vi "Title-Add.vi"(1 "Parameters":variant, 2 "String":string) -> (0 "Variant":variant)   [LabVIEW 2025]
doc: "Author: Scott Hannahs <sth@magnet.fsu.edu>\n\nThis software is licensed for use under the “MIT License\"\nCopyright (c) 2025 Scott Hannahs, sth@sth@magnet.sthnet.net\n\nPermission is hereby granted, free of charge, to any person obtaining a copy of this software and associated documentation files (the \"Software\"), to deal in the Software without restriction, including without limitation the rights to use, copy, modify, merge, publish, distribute, sublicense, and/or sell copies of the Software, and to permit persons to whom the Software is furnished to do so, subject to the following conditions: The above copyright notice and this permission notice shall be included in all copies or substantial portions of the Software.\n\nTHE SOFTWARE IS PROVIDED \"AS IS\", WITHOUT WARRANTY OF ANY KIND, EXPRESS OR IMPLIED, INCLUDING BUT NOT LIMITED TO THE WARRANTIES OF MERCHANTABILITY, FITNESS FOR A PARTICULAR PURPOSE AND NONINFRINGEMENT. IN NO EVENT SHALL THE AUTHORS OR COPYRIGHT HOLDERS BE LIABLE FOR ANY CLAIM, DAMAGES OR OTHER LIABILITY, WHETHER IN AN ACTION OF CONTRACT, TORT OR OTHERWISE, ARISING FROM, OUT OF OR IN CONNECTION WITH THE SOFTWARE OR THE USE OR OTHER DEALINGS IN THE SOFTWARE."
uses:
  Sub Controls/SystemCheckBox-resize.ctl
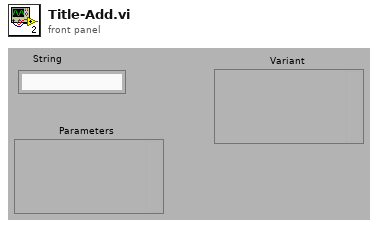
[diagram p1: front panel]
types:
  T1 = typedef "SystemCheckBox-resize.ctl" = bool
  T2 = typedef "Instrument Properties.ctl" = cluster{"Public":T3, "Private":T4}
  T3 = typedef "Public.ctl" = cluster{"Column Name":string[], "Trace Color":u32[]}
  T4 = typedef "Private.ctl" = cluster{"Path":path, "VI Refnum":T5, "Name":string, "# of Values":i32, "Scale Factors":dbl[], "Display":T1[], "Offset":dbl[]}
  T5 = typedef "Instrument Ref.ctl" = refnum<vi>
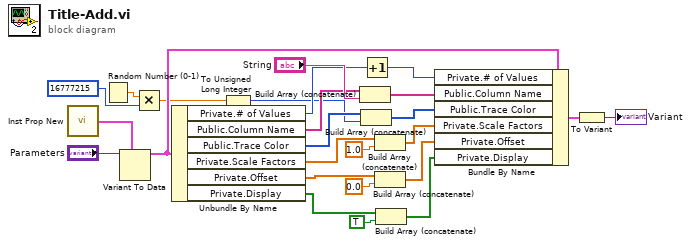
[diagram p0: block diagram]
diagram:
  n1 = call "Inst Prop New.vi"() -> ("Instrument Prop Out"=w23:T2)
  n2 = Random Number (0-1)() -> (number: 0 to 1=w14:dbl)
  n3 = Variant To Data(type=w23, Variant="Parameters") -> (data=w20:T2)  [unwired: 1 in, 1 out]
  n4 = Multiply(x=w14, y=u32 16777215) -> (x*y=w12:dbl)
  n5 = Unbundle By Name(w20) -> ("Private.# of Values"=w19:i32, "Public.Column Name"=w18:string[], "Public.Trace Color"=w16:u32[], "Private.Scale Factors"=w7:dbl[], "Private.Offset"=w1:dbl[], "Private.Display"=w6:T1[])
  n6 = To Unsigned Long Integer(number=w12) -> (unsigned 32bit integer=w11:u32)
  n7 = Build Array (concatenate)(w18, "String") -> (w21:string[])
  n8 = Build Array (concatenate)(w16, w11) -> (w15:u32[])
  n9 = Increment(x=w19) -> (x+1=w10:i32)
  n10 = Build Array (concatenate)(w7, 1.0) -> (w8:dbl[])
  n11 = Build Array (concatenate)(w1, 0.0) -> (w2:dbl[])
  n12 = Build Array (concatenate)(w6, T1 TRUE ("Display")) -> (w9:T1[])
  n13 = Bundle By Name(cluster=w20, "Private.# of Values"=w10, "Public.Column Name"=w21, "Public.Trace Color"=w15, "Private.Scale Factors"=w8, "Private.Offset"=w2, "Private.Display"=w9) -> (w17:T2)
  n14 = To Variant(anything=w17) -> (Variant=→"Variant":variant)
